vi "isValid FPGA Addon.vi"(8 "error in":errorcluster, 11 "FPGA Addon refnum in":T1=18446744073709551615 format="%.0x") -> (0 "error out":errorcluster, 3 "FPGA Addon refnum out":T1=18446744073709551615 format="%.0x")   [LabVIEW 2019, in "FPGA Addon Test Class.lvclass"]
uses:
  FPGA Addon Test Class.lvclass
  <vilib>/NI/NI VeriStand Advanced SysDef API/SysDef API/Advanced System Definition.lvlib
  Addon/Addon Shared/SubVIs/Constants.vi
  Addon/Addon Shared/FPGA Addon Shared.lvlib
  <vilib>/NI VeriStand/Custom Device API/Custom Device Item Ref.ctl
  <vilib>/NI VeriStand/Custom Device API/Custom Device API.lvlib
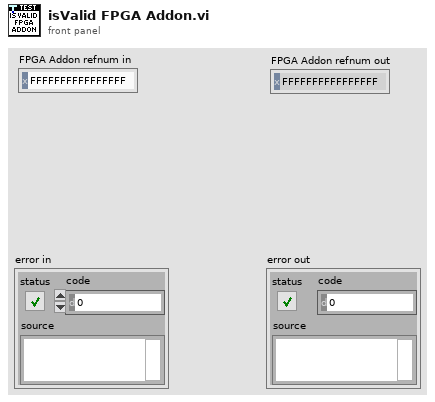
[diagram p1: front panel]
types:
  T1 = typedef "Custom Device API.lvlib/Custom Device Item Ref.ctl" = u64
  T2 = typedef "Advanced System Definition.lvlib/TreeItem.Info.ctl" = cluster{"Name":string, "Description":string, "GUID":string, "Is Channel":bool, "Channel":T3, "Is Waveform":bool, "Waveform":T5}
  T3 = typedef "Custom Device API.lvlib/Custom Device Channel.ctl" = cluster{"Type":T4, "Units":string, "Default Value":dbl, "Faultable":bool, "Scalable":bool}
  T4 = typedef "Custom Device API.lvlib/Custom Device Channel Type.ctl" = enum16{"Input", "Output"}
  T5 = typedef "Custom Device API.lvlib/Custom Device Waveform.ctl" = cluster{"Data Type":T6, "Units":string}
  T6 = typedef "Custom Device API.lvlib/Custom Device Waveform DataType.ctl" = enum16{"Double", "Complex Double"}
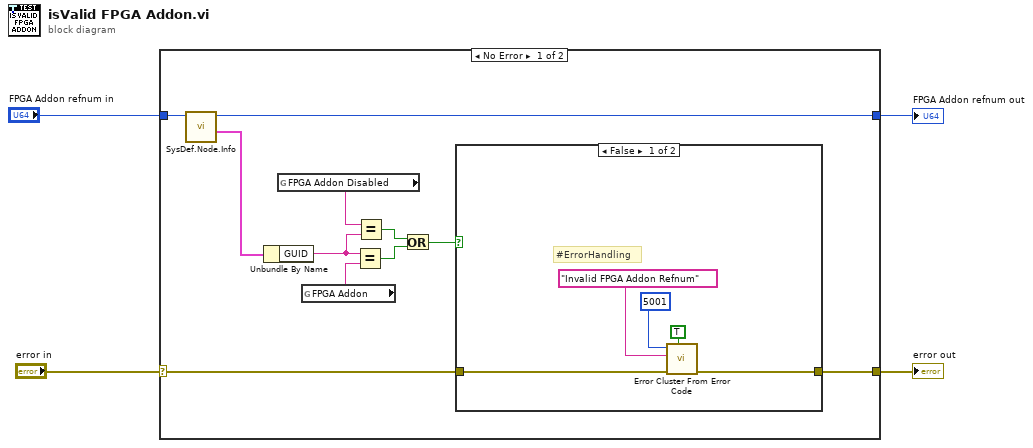
[diagram p0: block diagram]
diagram:
  n1 = case shown="No Error" "error in" {
    selector: "error in" -> [w6 w22]
    tunnel: "FPGA Addon refnum in" -> [w15 w23]
    tunnel: [w8 w23] -> w3
    tunnel: [w5 w22] -> w1
    frame No Error {
      n2 = call <vilib>:"SysDef.Node.Info.vi"("nodeID"=w15) -> ("Item Info"=w14:T2, "nodeID out"=w8:u64)  [unwired: 7 in, 2 out]
      n3 = Unbundle By Name(w14) -> ("GUID"=w12:string)
      n4 = global read "Constants.vi" "FPGA Addon Disabled"() -> (w11:string)
      n5 = global read "Constants.vi" "FPGA Addon"() -> (w13:string)
      n6 = Equal?(x=w12, y=w13) -> (x = y?=w10:bool)
      n7 = Equal?(x=w11, y=w12) -> (x = y?=w9:bool)
      n8 = Or(x=w9, y=w10) -> (x .or. y?=w7:bool)
      n9 = case shown="False" w7 {
        tunnel: w6 -> [w20 w21]
        tunnel: [w19 w21] -> w5
        frame False {
          # "#ErrorHandling"
          n10 = call <vilib>:"Error Cluster From Error Code.vi"("show call chain? (False)"=TRUE, "error in (no error)"=w20, "error message (\"\")"="Invalid FPGA Addon Refnum" ("error message (\"\")"), "error code (0)"=5001) -> ("error out"=w19:errorcluster)  [unwired: 5 in]
        }
        frame True {
        }
      }
    }
    frame Error {
    }
  }
  "error out" <- w1
  "FPGA Addon refnum out" <- w3
